vi "DIRECT SUMMING.vi"(0 "Image Data":dbl[][](array[numeric]), 1 "Fitting Results Save Path":string, 5 "Best Fit Parameters":dbl[](array[numeric]), 7 "File Num":u16, 9 "Fitting Type":u16(ring) items=["2D Gaussian", "2D Quadraple", "Double Gaussian", "Double Quadraple", "Triple Gaussian"], 11 "Two Cameras?":bool, 12 "Na / Rb":u16(ring) items=["Na", "Rb"]) -> (4 "XY Graph":cluster{dbl[], dbl[]}[](graph))   [LabVIEW 2015]
panel:
  out "Atom Number":dbl[](array[numeric])
  out "transposed array 3":dbl[][](array[numeric])
  out "transposed array 2":dbl[][](array[numeric])
  out "transposed array":dbl[][](array[numeric])
  out "appended array":dbl[](array[numeric])
  out "split 2":dbl
  out "split 1":dbl
  out "hbar in 10^-34 J.s":dbl
  out "Saturation Intensity in mW/cm^2":dbl
  out "Transition Angular Freq in THz":dbl
  out "Natural Linewidth in MHz":dbl
  in  "Experimental Parameters":T1
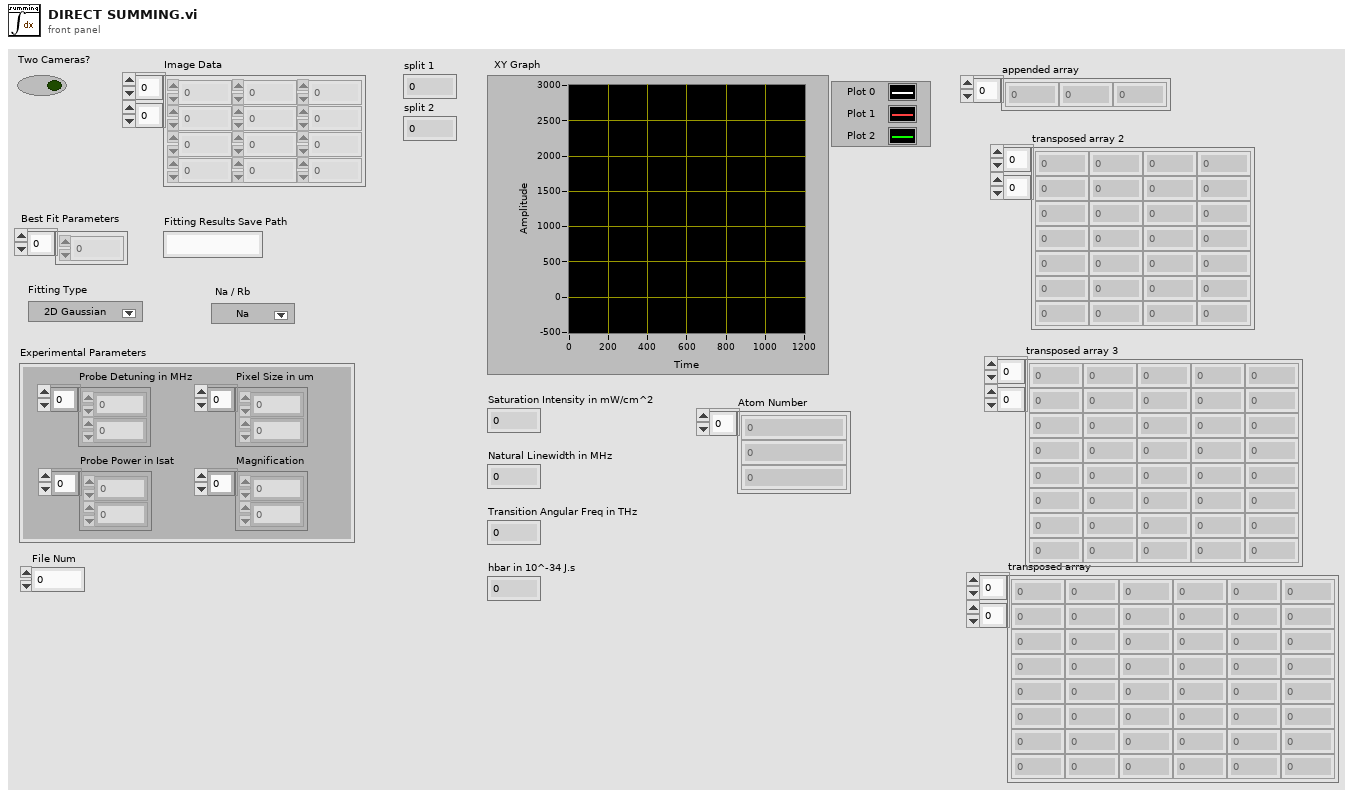
[diagram p1: front panel]
types:
  T1 = cluster{"Probe Detuning in MHz":dbl[], "Probe Power in Isat":dbl[], "Pixel Size in um":dbl[], "Magnification":dbl[]}
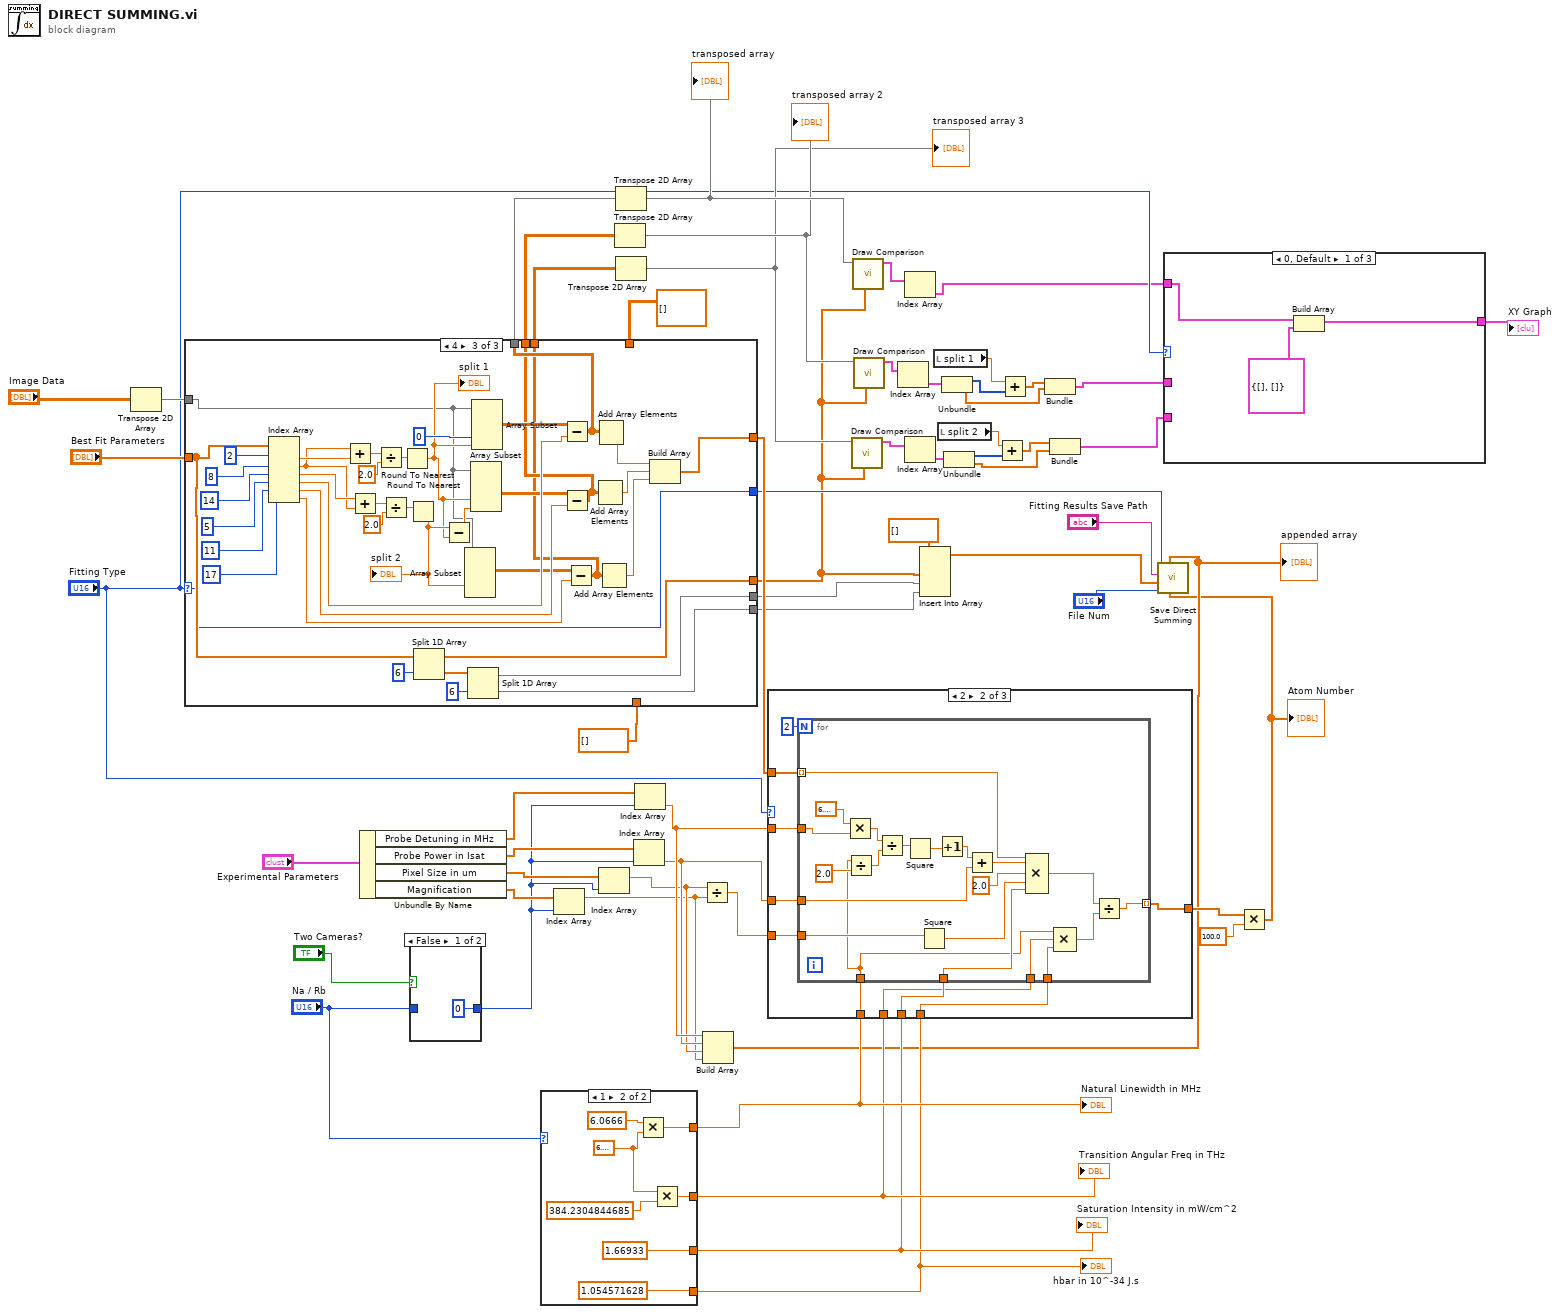
[diagram p0: block diagram]
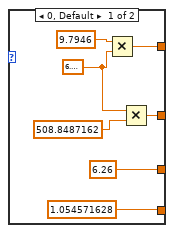
[diagram p3: hidden frame]
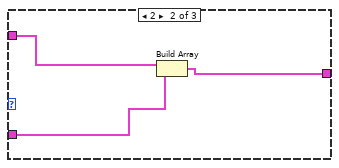
[diagram p4: hidden frame]
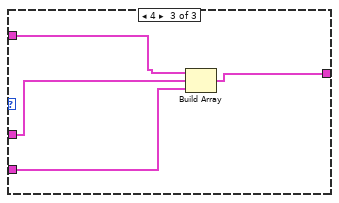
[diagram p5: hidden frame]
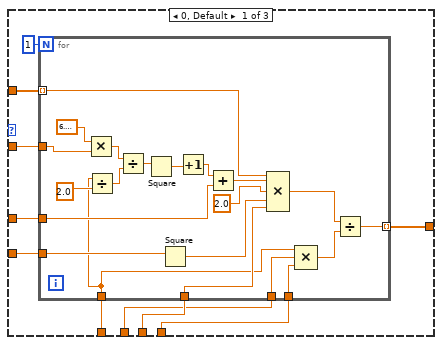
[diagram p6: hidden frame]
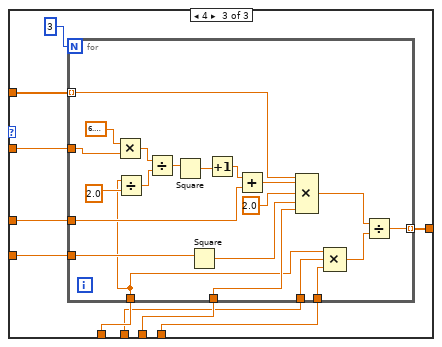
[diagram p7: hidden frame]
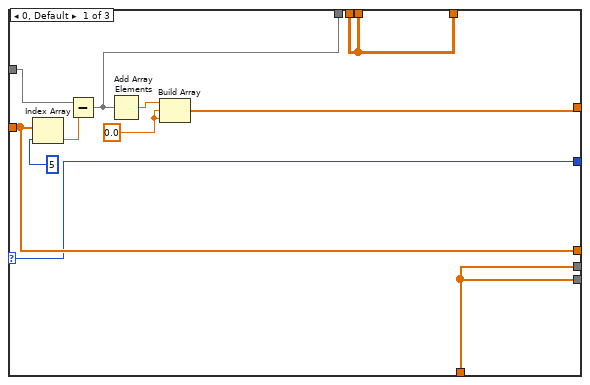
[diagram p8: hidden frame]
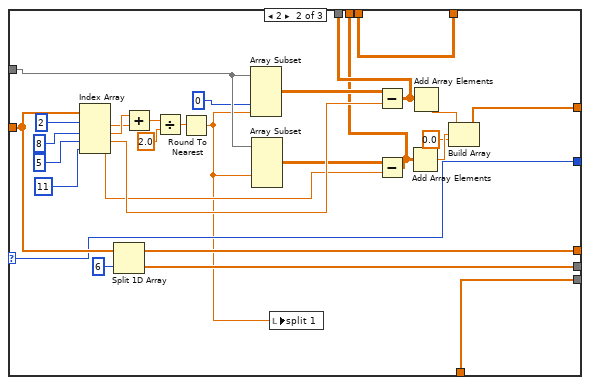
[diagram p9: hidden frame]
diagram:
  n1 = Transpose 2D Array(2D array="Image Data") -> (transposed array=w57:dbl[][])
  n2 = case shown="4" "Fitting Type" {
    selector: "Fitting Type" -> [w61 w75 w103]
    tunnel: w57 -> [w69 w90 w116]
    tunnel: "Best Fit Parameters" -> [w63 w80 w109]
    tunnel: [w66 w86 w111] -> w48
    tunnel: [w65 w73 w102] -> w55
    tunnel: [w64 w72 w101] -> w54
    tunnel: [w64 w81 w100] -> w53
    tunnel: dbl[][] [] -> [w64 w81 _]
    tunnel: [w63 w78 w107] -> w4
    tunnel: [w62 w77 w105] -> w29
    tunnel: dbl[] [] -> [w62 w76 _]
    tunnel: [w62 w76 w104] -> w28
    tunnel: [w61 w75 w103] -> w24
    frame 0, Default {
      w60 = 0.0 ("element")
      n3 = Index Array(array=w63, index=5) -> (element=w68:dbl)
      n4 = Subtract(x=w69, y=w68) -> (x-y=w65:dbl[][])
      n5 = Add Array Elements(numeric array=w65) -> (sum=w67:dbl)
      n6 = Build Array(w67, w60, w60) -> (w66:dbl[])
    }
    frame 2 {
      n7 = Index Array(array=w80, index #1=2 ("index"), index #2=8 ("index"), index #3=5 ("index"), index #4=11 ("index")) -> (element #1=w94:dbl, element #2=w95:dbl, element #3=w85:dbl, element #4=w84:dbl)
      n8 = Split 1D Array(array=w80, index=6) -> (first subarray=w78:dbl[], second subarray=w77:dbl[])
      n9 = Add(x=w95, y=w94) -> (x+y=w93:dbl)
      n10 = Divide(x=w93, y=2.0) -> (x/y=w91:dbl)
      n11 = Round To Nearest(number=w91) -> (nearest integer value=w74:dbl)
      n12 = Array Subset(array=w90, index (col)=0 ("index"), length (col)=w74) -> (w83:dbl[][])  [unwired: 2 in]
      n13 = Array Subset(array=w90, index (col)=w74) -> (w82:dbl[][])  [unwired: 3 in]
      n14 = local write "split 1"(w74) -> ()
      n15 = Subtract(x=w83, y=w85) -> (x-y=w73:dbl[][])
      n16 = Subtract(x=w82, y=w84) -> (x-y=w72:dbl[][])
      n17 = Add Array Elements(numeric array=w72) -> (sum=w87:dbl)
      n18 = Add Array Elements(numeric array=w73) -> (sum=w88:dbl)
      n19 = Build Array(w88, w87, 0.0 ("element")) -> (w86:dbl[])
    }
    frame 4 {
      n20 = Index Array(array=w109, index #1=2 ("index"), index #2=8 ("index"), index #3=14 ("index"), index #4=5 ("index"), index #5=11 ("index"), index #6=17 ("index")) -> (element #1=w136:dbl, element #2=w124:dbl, element #3=w125:dbl, element #4=w120:dbl, element #5=w119:dbl, element #6=w118:dbl)
      n21 = Add(x=w124, y=w136) -> (x+y=w135:dbl)
      n22 = Add(x=w125, y=w124) -> (x+y=w127:dbl)
      n23 = Divide(x=w135, y=2.0) -> (x/y=w133:dbl)
      n24 = Divide(x=w127, y=2.0) -> (x/y=w123:dbl)
      n25 = Round To Nearest(number=w133) -> (nearest integer value=w117:dbl)
      "split 1" <- w117
      n26 = Round To Nearest(number=w123) -> (nearest integer value=w121:dbl)
      "split 2" <- w121
      n27 = Split 1D Array(array=w109, index=6) -> (first subarray=w107:dbl[], second subarray=w106:dbl[])
      n28 = Subtract(x=w121, y=w117) -> (x-y=w122:dbl)
      n29 = Array Subset(array=w116, index (col)=w121) -> (w112:dbl[][])  [unwired: 3 in]
      n30 = Split 1D Array(array=w106, index=6) -> (first subarray=w105:dbl[], second subarray=w104:dbl[])
      n31 = Array Subset(array=w116, index (col)=w117, length (col)=w122) -> (w113:dbl[][])  [unwired: 2 in]
      n32 = Array Subset(array=w116, index (col)=0 ("index"), length (col)=w117) -> (w114:dbl[][])  [unwired: 2 in]
      n33 = Subtract(x=w114, y=w120) -> (x-y=w102:dbl[][])
      n34 = Subtract(x=w113, y=w119) -> (x-y=w101:dbl[][])
      n35 = Subtract(x=w112, y=w118) -> (x-y=w100:dbl[][])
      n36 = Add Array Elements(numeric array=w101) -> (sum=w130:dbl)
      n37 = Add Array Elements(numeric array=w102) -> (sum=w131:dbl)
      n38 = Add Array Elements(numeric array=w100) -> (sum=w115:dbl)
      n39 = Build Array(w131, w130, w115) -> (w111:dbl[])
    }
  }
  n40 = Unbundle By Name("Experimental Parameters") -> ("Probe Detuning in MHz"=w37:dbl[], "Probe Power in Isat"=w36:dbl[], "Pixel Size in um"=w35:dbl[], "Magnification"=w34:dbl[])
  n41 = case shown="False" "Two Cameras?" {
    tunnel: [u16 0 ("Na / Rb") w142] -> w6
    tunnel: "Na / Rb" -> [_ w142]
    frame False {
    }
    frame True {
    }
  }
  n42 = case shown="1" "Na / Rb" {
    tunnel: [w148 w150] -> w44
    tunnel: [w145 w151] -> w43
    tunnel: [6.26 ("element") 1.66933 ("element")] -> w42
    tunnel: [1.054571628 ("element") 1.054571628 ("element")] -> w41
    frame 0, Default {
      w147 = 6.283185307179586
      n43 = Multiply(x=9.7946 ("element"), y=w147) -> (x*y=w148:dbl)
      n44 = Multiply(x=w147, y=508.8487162 ("element")) -> (x*y=w145:dbl)
    }
    frame 1 {
      w155 = 6.283185307179586
      n45 = Multiply(x=6.0666 ("element"), y=w155) -> (x*y=w150:dbl)
      n46 = Multiply(x=w155, y=384.2304844685 ("element")) -> (x*y=w151:dbl)
    }
  }
  "Natural Linewidth in MHz" <- w44
  "Transition Angular Freq in THz" <- w43
  "Saturation Intensity in mW/cm^2" <- w42
  "hbar in 10^-34 J.s" <- w41
  n47 = Index Array(array=w34, index=w6) -> (element=w30:dbl)
  n48 = Index Array(array=w35, index=w6) -> (element=w31:dbl)
  n49 = Transpose 2D Array(2D array=w54) -> (transposed array=w50:dbl[][])
  "transposed array 2" <- w50
  n50 = Transpose 2D Array(2D array=w55) -> (transposed array=w51:dbl[][])
  "transposed array" <- w51
  n51 = Transpose 2D Array(2D array=w53) -> (transposed array=w49:dbl[][])
  "transposed array 3" <- w49
  n52 = Index Array(array=w36, index=w6) -> (element=w32:dbl)
  n53 = Index Array(array=w37, index=w6) -> (element=w33:dbl)
  n54 = Divide(x=w31, y=w30) -> (x/y=w45:dbl)
  n55 = Build Array(w33, w32, w31, w30) -> (w22:dbl[])
  "appended array" <- w22
  n56 = case shown="2" "Fitting Type" {
    tunnel: w48 -> [w165 w196 w227]
    tunnel: w33 -> [w164 w195 w219]
    tunnel: w32 -> [w162 w193 w225]
    tunnel: w45 -> [w161 w192 w224]
    tunnel: w44 -> [w163 w194 w226]
    tunnel: w43 -> [w158 w189 w221]
    tunnel: w42 -> [w160 w191 w223]
    tunnel: w41 -> [w159 w190 w222]
    tunnel: [w157 w188 w220] -> w40
    frame 0, Default {
      n57 = for {
        N: 1 -> [_]
        tunnel: w165 -> [w168] mode=indexing
        tunnel: w164 -> [w186]
        tunnel: w163 -> [w171]
        tunnel: w162 -> [w179]
        tunnel: w161 -> [w178]
        tunnel: w160 -> [w174]
        tunnel: w159 -> [w173]
        tunnel: w158 -> [w172]
        tunnel: [w167] -> w157 mode=indexing
        n58 = Multiply(x=6.283185307179586, y=w186) -> (x*y=w184:dbl)
        n59 = Divide(x=w171, y=2.0 ("x")) -> (x/y=w183:dbl)
        n60 = Divide(x=w184, y=w183) -> (x/y=w182:dbl)
        n61 = Square(x=w182) -> (x^2=w181:dbl)
        n62 = Square(x=w178) -> (x^2=w175:dbl)
        n63 = Increment(x=w181) -> (x+1=w180:dbl)
        n64 = Add(x=w180, y=w179) -> (x+y=w177:dbl)
        n65 = Compound Arithmetic op=MULTIPLY(w168, w177, 2.0 ("value"), w175, w174) -> (w170:dbl)
        n66 = Compound Arithmetic op=MULTIPLY(w171, w172, w173) -> (w169:dbl)
        n67 = Divide(x=w170, y=w169) -> (x/y=w167:dbl)
      }
    }
    frame 2 {
      n68 = for {
        N: 2 -> [_]
        tunnel: w196 -> [w199] mode=indexing
        tunnel: w195 -> [w217]
        tunnel: w194 -> [w202]
        tunnel: w193 -> [w210]
        tunnel: w192 -> [w209]
        tunnel: w191 -> [w205]
        tunnel: w190 -> [w204]
        tunnel: w189 -> [w203]
        tunnel: [w198] -> w188 mode=indexing
        n69 = Multiply(x=6.283185307179586, y=w217) -> (x*y=w215:dbl)
        n70 = Divide(x=w202, y=2.0 ("x")) -> (x/y=w214:dbl)
        n71 = Divide(x=w215, y=w214) -> (x/y=w213:dbl)
        n72 = Square(x=w213) -> (x^2=w212:dbl)
        n73 = Square(x=w209) -> (x^2=w206:dbl)
        n74 = Increment(x=w212) -> (x+1=w211:dbl)
        n75 = Add(x=w211, y=w210) -> (x+y=w208:dbl)
        n76 = Compound Arithmetic op=MULTIPLY(w199, w208, 2.0 ("value"), w206, w205) -> (w201:dbl)
        n77 = Compound Arithmetic op=MULTIPLY(w202, w203, w204) -> (w200:dbl)
        n78 = Divide(x=w201, y=w200) -> (x/y=w198:dbl)
      }
    }
    frame 4 {
      n79 = for {
        N: 3 -> [_]
        tunnel: w227 -> [w230] mode=indexing
        tunnel: w219 -> [w248]
        tunnel: w226 -> [w233]
        tunnel: w225 -> [w241]
        tunnel: w224 -> [w240]
        tunnel: w223 -> [w236]
        tunnel: w222 -> [w235]
        tunnel: w221 -> [w234]
        tunnel: [w229] -> w220 mode=indexing
        n80 = Multiply(x=6.283185307179586, y=w248) -> (x*y=w246:dbl)
        n81 = Divide(x=w233, y=2.0 ("x")) -> (x/y=w245:dbl)
        n82 = Divide(x=w246, y=w245) -> (x/y=w244:dbl)
        n83 = Square(x=w244) -> (x^2=w243:dbl)
        n84 = Square(x=w240) -> (x^2=w237:dbl)
        n85 = Increment(x=w243) -> (x+1=w242:dbl)
        n86 = Add(x=w242, y=w241) -> (x+y=w239:dbl)
        n87 = Compound Arithmetic op=MULTIPLY(w230, w239, 2.0 ("value"), w237, w236) -> (w232:dbl)
        n88 = Compound Arithmetic op=MULTIPLY(w233, w234, w235) -> (w231:dbl)
        n89 = Divide(x=w232, y=w231) -> (x/y=w229:dbl)
      }
    }
  }
  n90 = call "Draw Comparison.vi"("Best Fit Parameters"=w4, "Raw Data"=w49) -> ("Vertical Comparison"=w1:cluster{i32[], dbl[]}[])  [unwired: 7 in, 1 out]
  n91 = call "Draw Comparison.vi"("Best Fit Parameters"=w4, "Raw Data"=w51) -> ("Vertical Comparison"=w3:cluster{i32[], dbl[]}[])  [unwired: 7 in, 1 out]
  n92 = call "Draw Comparison.vi"("Best Fit Parameters"=w4, "Raw Data"=w50) -> ("Vertical Comparison"=w2:cluster{i32[], dbl[]}[])  [unwired: 7 in, 1 out]
  n93 = Index Array(array=w2) -> (element=w20:cluster{i32[], dbl[]})  [unwired: 1 in]
  n94 = Index Array(array=w3) -> (element=w18:cluster{i32[], dbl[]})  [unwired: 1 in]
  n95 = Index Array(array=w1) -> (element=w19:cluster{i32[], dbl[]})  [unwired: 1 in]
  n96 = Insert Into Array(array=dbl[] [], new element #1=w4, new element #2=w29, new element #3=w28) -> (w26:dbl[])  [unwired: 1 in]
  n97 = local read "split 1"() -> (w14:dbl)
  n98 = local read "split 2"() -> (w17:dbl)
  n99 = Unbundle(w20) -> (w15:i32[], w12:dbl[])
  n100 = Unbundle(w19) -> (w16:i32[], w11:dbl[])
  n101 = Add(x=w17, y=w16) -> (x+y=w10:dbl[])
  n102 = Add(x=w14, y=w15) -> (x+y=w13:dbl[])
  n103 = Bundle(w13, w12) -> (w9:cluster{dbl[], dbl[]})  [unwired: 1 in]
  n104 = Bundle(w10, w11) -> (w8:cluster{dbl[], dbl[]})  [unwired: 1 in]
  n105 = case shown="0, Default" "Fitting Type" {
    tunnel: w18 -> [w251 w254 w258]
    tunnel: w9 -> [_ w253 w257]
    tunnel: [w252 w255 w259] -> w46
    tunnel: w8 -> [_ _ w256]
    frame 0, Default {
      n106 = Build Array(w251, cluster{i32[], dbl[]} {[], []} ("element")) -> (w252:cluster{i32[], dbl[]}[])
    }
    frame 2 {
      n107 = Build Array(w254, w253) -> (w255:cluster{dbl[], dbl[]}[])
    }
    frame 4 {
      n108 = Build Array(w258, w257, w256) -> (w259:cluster{dbl[], dbl[]}[])
    }
  }
  "XY Graph" <- w46
  n109 = Multiply(x=w40, y=100.0 ("element")) -> (x*y=w21:dbl[])
  "Atom Number" <- w21
  n110 = call "Save Direct Summing.vi"("Direct Sum"=w21, "Experimental parameters"=w22, "Current File Num"="File Num", "Best Fit Parameters"=w26, "Fitting Results Save Path"="Fitting Results Save Path", "Fitting Type"=w24) -> ()  [unwired: 6 in]
